vi "Create.vi"(4 "TypeMap in":refnum<class "TypeMap.lvclass">, 6 "commandTimeout":i32=-1, 8 "error in (no error)":errorcluster, 10 "object in":refnum<class>, 11 "SqlMapper in":refnum<class "SqlMapper.lvclass">) -> (0 "error out":errorcluster, 1 "id":i32, 2 "object out":refnum<class>, 3 "SqlMapper out":refnum<class "SqlMapper.lvclass">)   [LabVIEW 2020, in "ORM_API.lvlib"]
doc: "NSERT a single entities."
uses:
  ORM_API.lvlib
  <vilib>/Viviota/shared/ORM.lvlibp/ORM/TypeMap/TypeMap.lvclass
  <vilib>/Viviota/shared/ORM.lvlibp/ORM/SqlMapper/SqlMapper.lvclass
  <userlib>/_OpenG.lib/lvdata/lvdata.llb/LVOOP Is Default Value__ogtk.vi
  <vilib>/Viviota/shared/ORM.lvlibp/ORM/TypeMap/Read TypeMap.vi
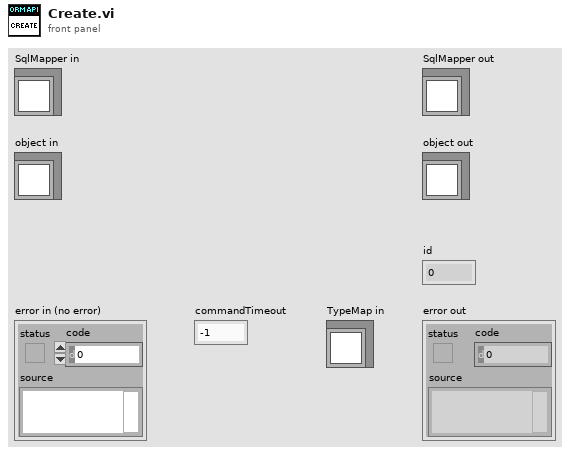
[diagram p1: front panel]
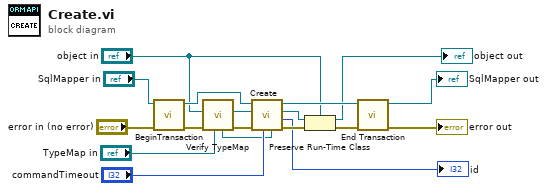
[diagram p0: block diagram]
diagram:
  n1 = call-dynamic "BeginTransaction.vi"("error in (no error)"="error in (no error)", "SqlMapper in"="SqlMapper in") -> ("error out"=w12:errorcluster, "SqlMapper out"=w14:refnum<class "SqlMapper.lvclass">)  [unwired: 8 in]
  n2 = call "Verify TypeMap.vi"("TypeMap in"="TypeMap in", "error in (no error)"=w12, "Type in"="object in") -> ("error out"=w10:errorcluster, "Type out"=w18:refnum<class>, "TypeMap out"=w7:refnum<class "TypeMap.lvclass">)  [unwired: 6 in]
  n3 = call-dynamic "Create.vi"("TypeMap in"=w7, "commandTimeout"="commandTimeout", "error in (no error)"=w10, "object in"=w18, "SqlMapper in"=w14) -> ("error out"=w9:errorcluster, "id"=→"id":i32, "object out"=w3:refnum<class>, "SqlMapper out"=w16:refnum<class "SqlMapper.lvclass">)  [unwired: 3 in]
  n4 = Preserve Run-Time Class(object in=w3, error in=w9, 2:"object in") -> (object out=→"object out":refnum<class>, error out=w4:errorcluster)
  n5 = call <vilib>:"End Transaction.vi"("error in (no error)"=w4, "SqlMapper in"=w16) -> ("error out"=→"error out":errorcluster, "SqlMapper out"=→"SqlMapper out":refnum<class "SqlMapper.lvclass">)  [unwired: 8 in]
